vi "Update Token.vi"(7 "Endpoint element key":string, 8 "error in (no error)":errorcluster, 9 "Value":string, 10 "Token element":T1, 11 "OAuthAccessToken in":refnum<class "OAuthAccessToken.lvclass">) -> (0 "error out":errorcluster, 3 "OAuthAccessToken out":refnum<class "OAuthAccessToken.lvclass">)   [LabVIEW 2013, in "OAuthAccessToken.lvclass"]
uses:
  OAuthAccessToken.lvclass
  OAuth2 Token Element -- enum.ctl
  OAuthAccessToken.lvclass/OAuthAccessToken.ctl
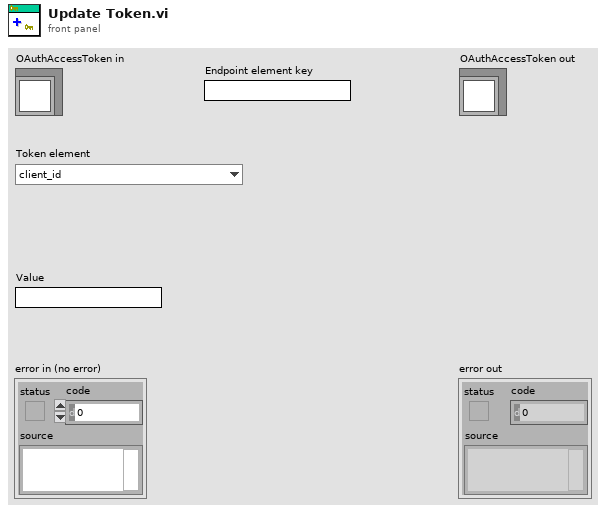
[diagram p1: front panel]
types:
  T1 = typedef "OAuthAccessToken.lvclass/OAuth2 Token Element -- enum.ctl" = enum16{"client_id", "client_secret", "response_type", "scope", "redirect_uri", "error", "error_description", "error_uri", "grant_type", "code", "access_token", "token_type", "expires_in", "username", "password", "refresh_token", "endpoint element"}
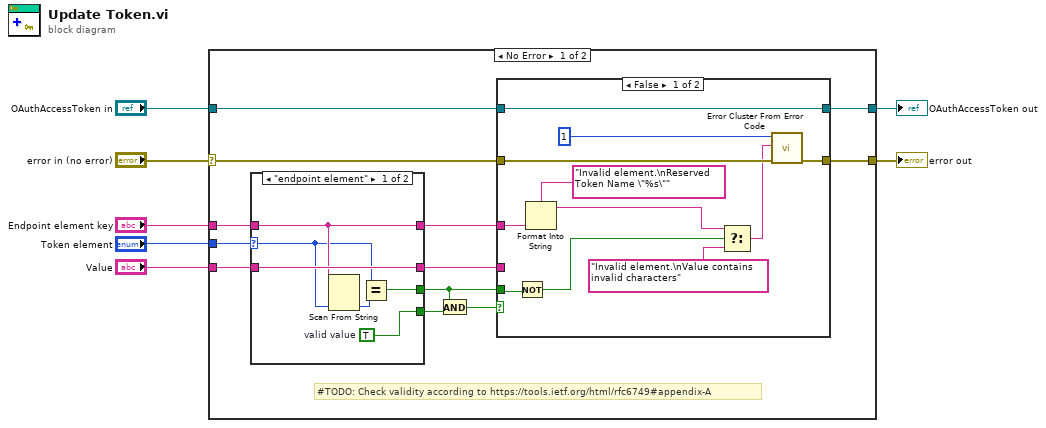
[diagram p0: block diagram]
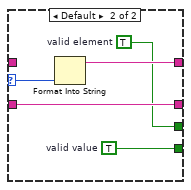
[diagram p2: hidden frame]
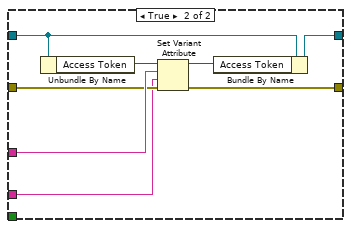
[diagram p3: hidden frame]
diagram:
  n1 = case shown="No Error" "error in (no error)" {
    selector: "error in (no error)" -> [w16 w51]
    tunnel: [w15 w51] -> w6
    tunnel: [w18 w50] -> w4
    tunnel: "OAuthAccessToken in" -> [w19 w50]
    tunnel: "Token element" -> [w14 _]
    tunnel: "Endpoint element key" -> [w13 _]
    tunnel: "Value" -> [w12 _]
    frame No Error {
      # "#TODO: Check validity according to https://tools.ietf.org/html/rfc6749#appendix-A"
      n2 = case shown="\"endpoint element\"" w14 {
        selector: w14 -> [w22 w29]
        tunnel: [w24 w30] -> w17
        tunnel: w13 -> [w24 _]
        tunnel: w12 -> [w25 w28]
        tunnel: [w25 w28] -> w11
        tunnel: [w20 w27] -> w9
        tunnel: [w21 w26] -> w8
        frame "endpoint element" {
          w20 = TRUE  # valid value
          n3 = Scan From String(input string=w24, default 1=w22) -> (output 1=w23:T1)  [unwired: 3 in, 3 out]
          n4 = Equal?(x=w22, y=w23) -> (x = y?=w21:bool)
        }
        frame Default {
          w26 = TRUE  # valid element
          w27 = TRUE  # valid value
          n5 = Format Into String(w29) -> (resulting string=w30:string)  [unwired: 3 in, 1 out]
        }
      }
      n6 = And(x=w8, y=w9) -> (x .and. y?=w10:bool)
      n7 = case shown="False" w10 {
        tunnel: w19 -> [w41 w49]
        tunnel: [w41 w48] -> w18
        tunnel: w17 -> [w33 w45]
        tunnel: w16 -> [w40 w44]
        tunnel: [w39 w43] -> w15
        tunnel: w11 -> [_ w42]
        tunnel: w8 -> [w37 _]
        frame False {
          n8 = Not(x=w37) -> (.not. x?=w34:bool)
          n9 = Format Into String(format string="Invalid element.\nReserved Token Name \"%s\"" ("error message (\"\")"), w33) -> (resulting string=w32:string)  [unwired: 2 in, 1 out]
          n10 = Select(t=w32, s=w34, f="Invalid element.\nValue contains invalid characters" ("error message (\"\")")) -> (s? t:f=w36:string)
          n11 = call <vilib>:"Error Cluster From Error Code.vi"("error in (no error)"=w40, "error message (\"\")"=w36, "error code (0)"=1) -> ("error out"=w39:errorcluster)  [unwired: 6 in]
        }
        frame True {
          n12 = Unbundle By Name(w49) -> ("Access Token"=w47:variant)
          n13 = Set Variant Attribute(Variant=w47, name=w45, value=w42, error in=w44) -> (Variant out=w46:variant, error out=w43:errorcluster)  [unwired: 1 out]
          n14 = Bundle By Name(cluster=w49, "Access Token"=w46) -> (w48:refnum<class "OAuthAccessToken.lvclass">)
        }
      }
    }
    frame Error {
    }
  }
  "error out" <- w6
  "OAuthAccessToken out" <- w4
